vi "Initialize All Structures (uSMC).vi"(8 "error in":errorcluster, 10 "axis":i32, 11 "Visa array in":refnum<visa-resource-name>[](array[refnum])) -> (0 "error out":errorcluster, 3 "Visa array out":refnum<visa-resource-name>[](array[refnum]))   [LabVIEW 2010, in "SignalWriterMH110203USBStepperMotor.lvclass"]
uses:
  SignalWriterMH110203USBStepperMotor.lvclass
  Get State Control (uSMC).ctl
  class_data.vi
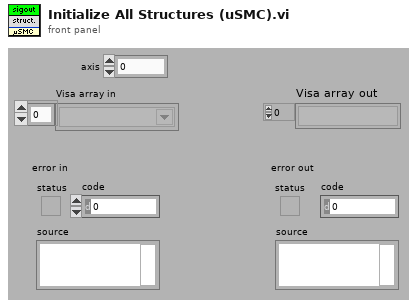
[diagram p1: front panel]
types:
  T1 = typedef "SignalWriterMH110203USBStepperMotor.lvclass/Get State Control (uSMC).ctl" = cluster{"Current Posistion":dbl, "CW/CCW":bool, "Speed":u16, "Temperature":dbl, "Power":u16, "Limit Switch 1":bool, "Limit Switch 2":bool, "After Reset":bool, "Step":u8, "Backlash":bool, "RT Error":bool, "RT State":bool, "Sync In":bool, "Sync Out":bool, "Ext Disconnect":bool, "Usb Powered":bool, "Voltage":dbl, "Working":bool, "SM Position in Encoder Units":i32, "Encoder Current Position":i32}
  T2 = typedef "SignalWriterMH110203USBStepperMotor.lvclass/GoTo Control (uSMC).ctl" = cluster{"Step motor ID":string, "SMname":string, "Backlash":u16, "wait for input sygnal to start":bool, "use slow start/stop":bool, "units name":string, "Maximum speed":dbl, "speed":dbl, "step":u8, "point 1 ticks":i32, "point 2 ticks":i32, "point 1 units":dbl, "point 2 units":dbl, "Limit Switch standoff":dbl, "Zero Value":dbl, "Destination Position":dbl, "force backlash":bool, "power off when stop":bool, "POff delay":dbl, "positioner name":string, "R, Ohm":dbl, "I, mA":dbl, "Positioner's Type":u16, "Reset Direction":bool, "Manufacturer":string, "Model":string, "Scheme":string, "FirmwareVer":string}
  T3 = typedef "SignalWriterMH110203USBStepperMotor.lvclass/Set Parameters (uSMC).ctl" = cluster{"Acceleration Time":u8, "Deceleration Time":u8, "Reduce Current Timeout":u16, "Buttons Timeout 1":u16, "Buttons Timeout 2":u16, "Buttons Timeout 3":u16, "Buttons Timeout 4":u16, "Buttons Timeout Reset":u16, "Buttons Timeout DblClick":u16, "Reset Speed":u16, "Buttons Speed 1":u16, "Buttons Speed 2":u16, "Buttons Speed 3":u16, "Buttons Speed 4":u16, "Max Backlash":u16, "Start Pos":i32, "RTdelta":u16, "RTMinError":u16, "Maximum Temperature":u16, "Sync Duration":u8, "Backlash Speed":u16, "EncVSCP":u8, "Steps Per Revolution":i32, "Encoder Pulses Per Rev-on":i32}
  T4 = cluster{"Cur Pos Units":dbl, "Set Cur Pos units":dbl, "Lo Limit Units":dbl, "Hi Limit Units":dbl, "Cur Pos Ticks":i32, "Set Cur Pos ticks":i32, "Lo Limit Ticks":i32, "Hi Limit Ticks":i32, "Minimal Value":dbl, "Maximal Value":dbl}[]
  T5 = typedef "SignalWriterMH110203USBStepperMotor.lvclass/Mode Control (uSMC).ctl" = cluster{"Turn Buttons Off":bool, "Reduce Current":bool, "Power Off and Make a Whole Step":bool, "Emergency Power Off":bool, "Limit Switch 1 True State":bool, "Limit Switch 2 True State":bool, "Rotary Transducer TRUE State":bool, "Swap Limit Switches":bool, "Limit Switch 1 Operation Enabled":bool, "Limit Switch 2 Operation Enabled":bool, "Rotary Transducer Operation Enabled":bool, "Rotary Transducer Operation Select":bool, "Button 1 True State":bool, "Button 2 True State":bool, "Swap Buttons":bool, "Reset Rotary Transducer Check Positions":bool, "Output Syncronization Enabled":bool, "Reset Output Sync Count":bool, "Sync Operation":bool, "Sync Count":u32, "Power":bool, "Invert Sync Polarity":bool, "Use Encoder":bool, "Invert Encoder Direction":bool, "Reset Encoder To 0":bool, "Reset SM Enc Pos to Enc Pos":bool}
  T6 = cluster{"Cur Pos Units":dbl, "Set Cur Pos units":dbl, "Lo Limit Units":dbl, "Hi Limit Units":dbl, "Cur Pos Ticks":i32, "Set Cur Pos ticks":i32, "Lo Limit Ticks":i32, "Hi Limit Ticks":i32, "Minimal Value":dbl, "Maximal Value":dbl}
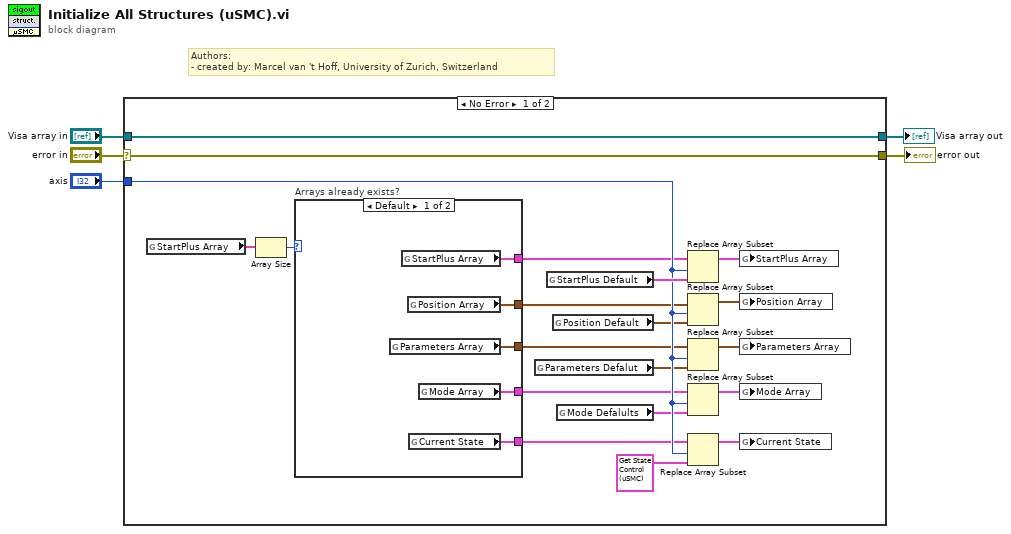
[diagram p0: block diagram]
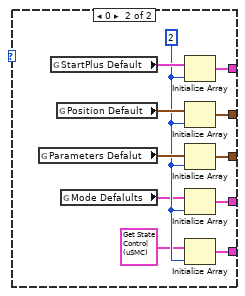
[diagram p2: hidden frame]
diagram:
  # "Authors: \n- created by: Marcel van 't Hoff, University of Zurich, Switzerland"
  n1 = case shown="No Error" "error in" {
    selector: "error in" -> [w25 w42]
    tunnel: "Visa array in" -> [w24 w43]
    tunnel: [w25 w42] -> w3
    tunnel: [w24 w43] -> w2
    tunnel: "axis" -> [w21 _]
    frame No Error {
      n2 = global read "class_data.vi" "StartPlus Array"() -> (w12:T2[])
      n3 = Array Size(array=w12) -> (size(s)=w11:i32)
      n4 = case "Arrays already exists?" shown="Default" w11 {
        tunnel: [w30 w40] -> w10
        tunnel: [w29 w38] -> w9
        tunnel: [w28 w33] -> w8
        tunnel: [w27 w32] -> w7
        tunnel: [w26 w31] -> w6
        frame Default {
          n5 = global read "class_data.vi" "Parameters Array"() -> (w28:T3[])
          n6 = global read "class_data.vi" "StartPlus Array"() -> (w30:T2[])
          n7 = global read "class_data.vi" "Position Array"() -> (w29:T4)
          n8 = global read "class_data.vi" "Current State"() -> (w26:T1[])
          n9 = global read "class_data.vi" "Mode Array"() -> (w27:T5[])
        }
        frame 0 {
          w36 = 2 ("dimension size")
          n10 = global read "class_data.vi" "Parameters Defalut"() -> (w37:T3)
          n11 = global read "class_data.vi" "StartPlus Default"() -> (w41:T2)
          n12 = global read "class_data.vi" "Position Default"() -> (w39:T6)
          n13 = global read "class_data.vi" "Mode Defalults"() -> (w35:T5)
          n14 = Initialize Array(w41, w36) -> (w40:T2[])
          n15 = Initialize Array(w39, w36) -> (w38:T4)
          n16 = Initialize Array(w37, w36) -> (w33:T3[])
          n17 = Initialize Array(w35, w36) -> (w32:T5[])
          n18 = Initialize Array(T1 {"Current Posistion"=0.0, "CW/CCW"=FALSE, "Speed"=0, "Temperature"=0.0, "Power"=0, "Limit Switch 1"=FALSE, "Limit Switch 2"=FALSE, "After Reset"=FALSE, "Step"=0, "Backlash"=FALSE, "RT Error"=FALSE, "RT State"=FALSE, "Sync In"=FALSE, "Sync Out"=FALSE, "Ext Disconnect"=FALSE, "Usb Powered"=FALSE, "Voltage"=0.0, "Working"=FALSE, "SM Position in Encoder Units"=0, "Encoder Current Position"=0} ("State cluster"), w36) -> (w31:T1[])
        }
      }
      n19 = global read "class_data.vi" "Parameters Defalut"() -> (w17:T3)
      n20 = global read "class_data.vi" "StartPlus Default"() -> (w23:T2)
      n21 = global read "class_data.vi" "Position Default"() -> (w20:T6)
      n22 = global read "class_data.vi" "Mode Defalults"() -> (w18:T5)
      n23 = Replace Array Subset(array=w10, new element=w23, index=w21) -> (w22:T2[])
      n24 = Replace Array Subset(array=w9, new element=w20, index=w21) -> (w16:T4)
      n25 = Replace Array Subset(array=w8, new element=w17, index=w21) -> (w15:T3[])
      n26 = Replace Array Subset(array=w7, new element=w18, index=w21) -> (w14:T5[])
      n27 = Replace Array Subset(array=w6, new element=T1 {"Current Posistion"=0.0, "CW/CCW"=FALSE, "Speed"=0, "Temperature"=0.0, "Power"=0, "Limit Switch 1"=FALSE, "Limit Switch 2"=FALSE, "After Reset"=FALSE, "Step"=0, "Backlash"=FALSE, "RT Error"=FALSE, "RT State"=FALSE, "Sync In"=FALSE, "Sync Out"=FALSE, "Ext Disconnect"=FALSE, "Usb Powered"=FALSE, "Voltage"=0.0, "Working"=FALSE, "SM Position in Encoder Units"=0, "Encoder Current Position"=0} ("State cluster"), index=w21) -> (w13:T1[])
      n28 = global write "class_data.vi" "StartPlus Array"(w22) -> ()
      n29 = global write "class_data.vi" "Position Array"(w16) -> ()
      n30 = global write "class_data.vi" "Parameters Array"(w15) -> ()
      n31 = global write "class_data.vi" "Mode Array"(w14) -> ()
      n32 = global write "class_data.vi" "Current State"(w13) -> ()
    }
    frame Error {
    }
  }
  "Visa array out" <- w2
  "error out" <- w3
